vi "Read Waveform Preamble.vi"(0 "Instrument Handle In":i32, 5 "Source":i32(ring) items=["Input Channel 1", "Input Channel 2", "Input Channel 3", "Input Channel 4", "Calc Channel 1", "Calc Channel 2", "Calc Channel 3", "Calc Channel 4", "Ref Channel 1", "Ref Channel 2", "Ref Channel 3", "Ref Channel 4"], 11 "error in":errorcluster) -> (2 "Voltage Offset":dbl, 3 "Voltage Interval":dbl, 4 "Instrument Handle Out":i32, 6 "Type":i32=1, 8 "Points":u32=100, 10 "Acquisition Count":i32=1, 13 "Time Offset":dbl, 14 "Time Interval":dbl=9.99999993922529e-09, 15 "error out":errorcluster)   [LabVIEW 2020, in "ZTScopeM.lvlib"]
doc: "Query the selected channel's preamble. The preamble contains all the information necessary to retrieve and interpret a waveform readback."
uses:
  ZTScopeM.lvlib
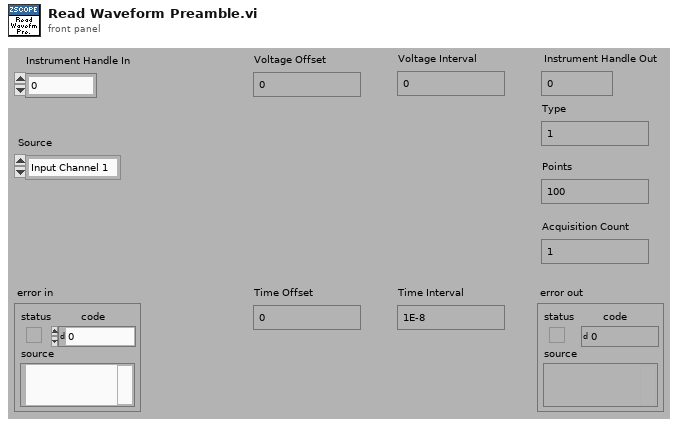
[diagram p1: front panel]
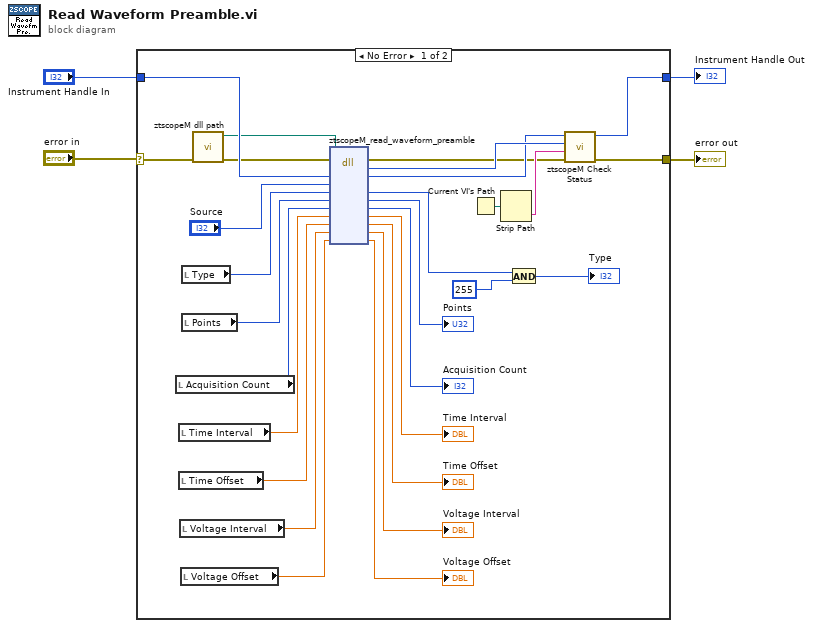
[diagram p0: block diagram]
diagram:
  n1 = case shown="No Error" "error in" {
    selector: "error in" -> [w8 w34]
    tunnel: [w15 w34] -> w1
    tunnel: "Instrument Handle In" -> [w32 w33]
    tunnel: [w14 w33] -> w3
    frame No Error {
      n2 = local read "Acquisition Count"() -> (w27:i32)
      n3 = local read "Time Interval"() -> (w25:dbl)
      n4 = local read "Time Offset"() -> (w23:dbl)
      n5 = local read "Voltage Interval"() -> (w9:dbl)
      n6 = local read "Voltage Offset"() -> (w21:dbl)
      n7 = local read "Type"() -> (w30:i32)
      n8 = local read "Points"() -> (w29:u32)
      n9 = call "ztscopeM dll path.vi"("error in (no error)"=w8) -> ("error out"=w6:errorcluster, "<instrument>.dll path"=w7:path)  [unwired: 9 in]
      n10 = dll-call lib="C:/Program Files (x86)/National Instruments/LabVIEW 2013/instr.lib/ztscopem/ztscopeM.dll" fn="ztscopeM_read_waveform_preamble"(path in=w7, error in=w6, "instrumentHandle"=w32, "source"="Source", "type"=w30, "points"=w29, "acquisitionCount"=w27, "timeInterval"=w25, "timeOffset"=w23, "voltageInterval"=w9, "voltageOffset"=w21) -> (error out=w5:errorcluster, w17:i32, "instrumentHandle"=w16:i32, "type"=w12:i32, "points"=→"Points":u32, "acquisitionCount"=→"Acquisition Count":i32, "timeInterval"=→"Time Interval":dbl, "timeOffset"=→"Time Offset":dbl, "voltageInterval"=→"Voltage Interval":dbl, "voltageOffset"=→"Voltage Offset":dbl)  [unwired: 2 in, 1 out]
      n11 = Current VI's Path() -> (path=w19:path)
      n12 = Strip Path(path=w19) -> (name=w18:string)  [unwired: 1 out]
      n13 = And(x=w12, y=255) -> (x .and. y?=→"Type":i32)
      n14 = call "ztscopeM Check Status.vi"("error in"=w5, "name of VI"=w18, "status (return code)"=w17, "instrument handle in"=w16) -> ("error out"=w15:errorcluster, "instrument handle out"=w14:i32)  [unwired: 2 in]
    }
    frame Error {
    }
  }
  "Instrument Handle Out" <- w3
  "error out" <- w1
